vi "w.vi"(8 "error in (no error)":errorcluster, 11 "Completion Ack Msg in":refnum<class "Completion Notification Msg.lvclass">) -> (0 "error out":errorcluster, 2 "Current Execution Count":u32, 3 "Completion Ack Msg out":refnum<class "Completion Notification Msg.lvclass">)   [LabVIEW 2021, in "Async Methods Actor.lvlib" / "Completion Notification Msg.lvclass"]
uses:
  Completion Notification Msg.lvclass
  Completion Notification Msg.lvclass/Completion Notification Msg.ctl
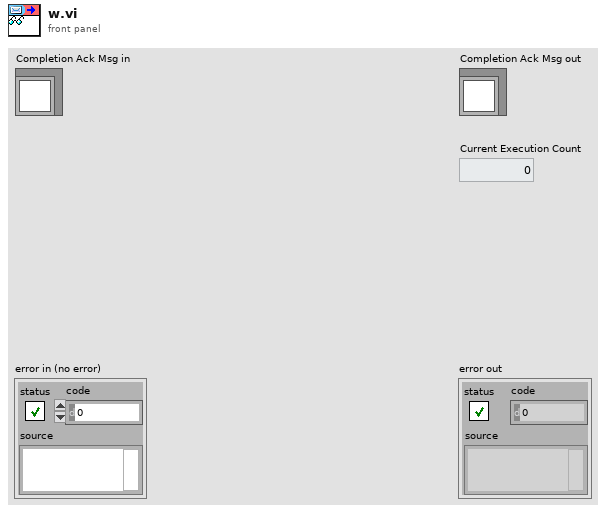
[diagram p1: front panel]
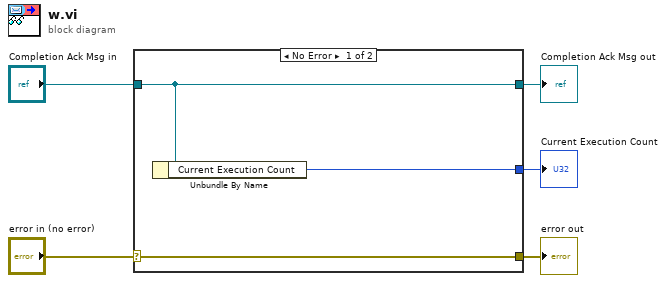
[diagram p0: block diagram]
diagram:
  n1 = case shown="No Error" "error in (no error)" {
    selector: "error in (no error)" -> [w8 w9]
    tunnel: [w8 w9] -> w4
    tunnel: [w7 w10] -> w2
    tunnel: "Completion Ack Msg in" -> [w7 w10]
    tunnel: [w6 _] -> w1
    frame No Error {
      n2 = Unbundle By Name(w7) -> ("Current Execution Count"=w6:u32)
    }
    frame Error {
    }
  }
  "error out" <- w4
  "Completion Ack Msg out" <- w2
  "Current Execution Count" <- w1
